vi "testMiror.vi"() -> ()   [LabVIEW 2020]
uses:
  ALPAO/ALPAO.lvclass
  mirror.lvclass
panel:
  in  "stop":bool
  in  "serial":string="alpaoLSDM88-25-001"
  in  "value":dbl[](array[numeric])
  out "offset":dbl[](array[numeric])
  out "NbActuator":i32
  out "error out":errorcluster
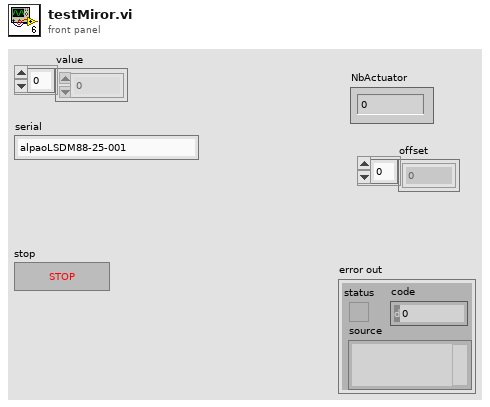
[diagram p1: front panel]
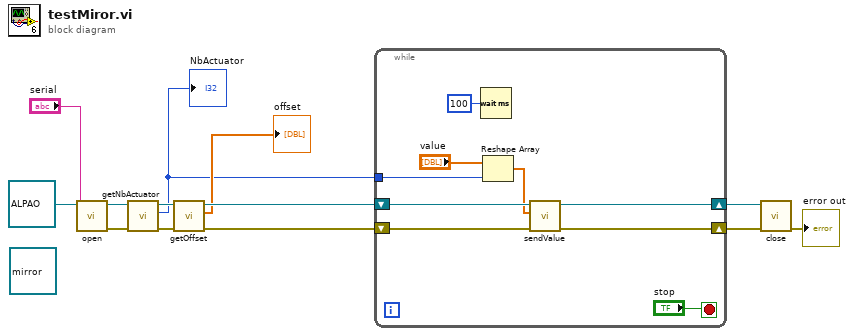
[diagram p0: block diagram]
diagram:
  (unwired) refnum<class "mirror.lvclass"> refnum ("mirror.lvclass")
  n1 = call-dynamic "open.vi"("serial"="serial", "ALPAO in"=refnum<class "ALPAO.lvclass"> refnum ("ALPAO.lvclass")) -> ("error out"=w6:errorcluster, "ALPAO out"=w13:refnum<class "ALPAO.lvclass">)  [unwired: 8 in]
  n2 = call-dynamic "getNbActuator.vi"("error in (no error)"=w6, "ALPAO in"=w13) -> ("error out"=w7:errorcluster, "NbActuator"=w2:i32, "ALPAO out"=w12:refnum<class "ALPAO.lvclass">)  [unwired: 7 in]
  "NbActuator" <- w2
  n3 = call-dynamic "getOffset.vi"("error in (no error)"=w7, "ALPAO in"=w12) -> ("error out"=w8:errorcluster, "offset"=→"offset":dbl[], "ALPAO out"=w11:refnum<class "ALPAO.lvclass">)  [unwired: 7 in]
  n4 = while {
    tunnel: w2 -> [w16]
    shift-right: [w21] -> w10
    shift-left: w11 -> [w22]
    shift-right: [w20] -> w9
    shift-left: w8 -> [w19]
    stop <- "stop" stop-if-true
    n5 = Wait (ms)(milliseconds to wait=u32 100) -> ()  [unwired: 1 out]
    n6 = Reshape Array("value", w16) -> (w17:dbl[])
    n7 = call-dynamic "sendValue.vi"("error in (no error)"=w19, "tabCom"=w17, "ALPAO in"=w22) -> ("error out"=w20:errorcluster, "ALPAO out"=w21:refnum<class "ALPAO.lvclass">)  [unwired: 7 in]
  }
  n8 = call-dynamic "close.vi"("error in (no error)"=w9, "ALPAO in"=w10) -> ("error out"=→"error out":errorcluster)  [unwired: 8 in, 1 out]
